vi "Power ASIC EEPROM Read.vi"(8 "error in (no error)":errorcluster) -> (0 "error out":errorcluster, 2 "results string":string, 3 "Cluster":T1)   [LabVIEW 2010]
panel:
  in  "Silicon Revision":enum16{"Rev 1-2", "Rev 3 +"}(ring)
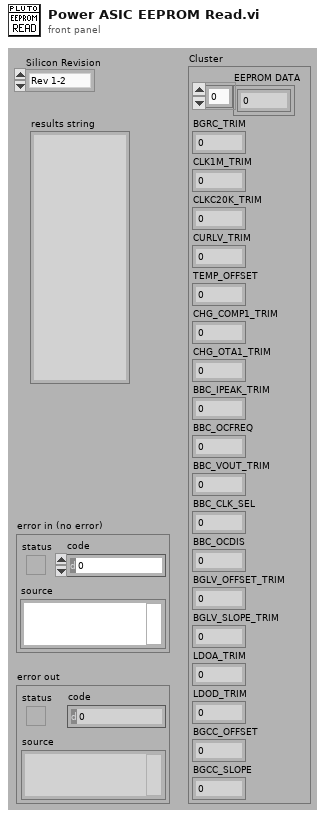
[diagram p1: front panel]
types:
  T1 = cluster{"EEPROM DATA":u32[], "BGRC_TRIM":u16, "CLK1M_TRIM":u16, "CLKC20K_TRIM":u16, "CURLV_TRIM":u16, "TEMP_OFFSET":u16, "CHG_COMP1_TRIM":u16, "CHG_OTA1_TRIM":u16, "BBC_IPEAK_TRIM":u16, "BBC_OCFREQ":u16, "BBC_VOUT_TRIM":u16, "BBC_CLK_SEL":u16, "BBC_OCDIS":u16, "BGLV_OFFSET_TRIM":u16, "BGLV_SLOPE_TRIM":u16, "LDOA_TRIM":u16, "LDOD_TRIM":u16, "BGCC_OFFSET":u16, "BGCC_SLOPE":u16}
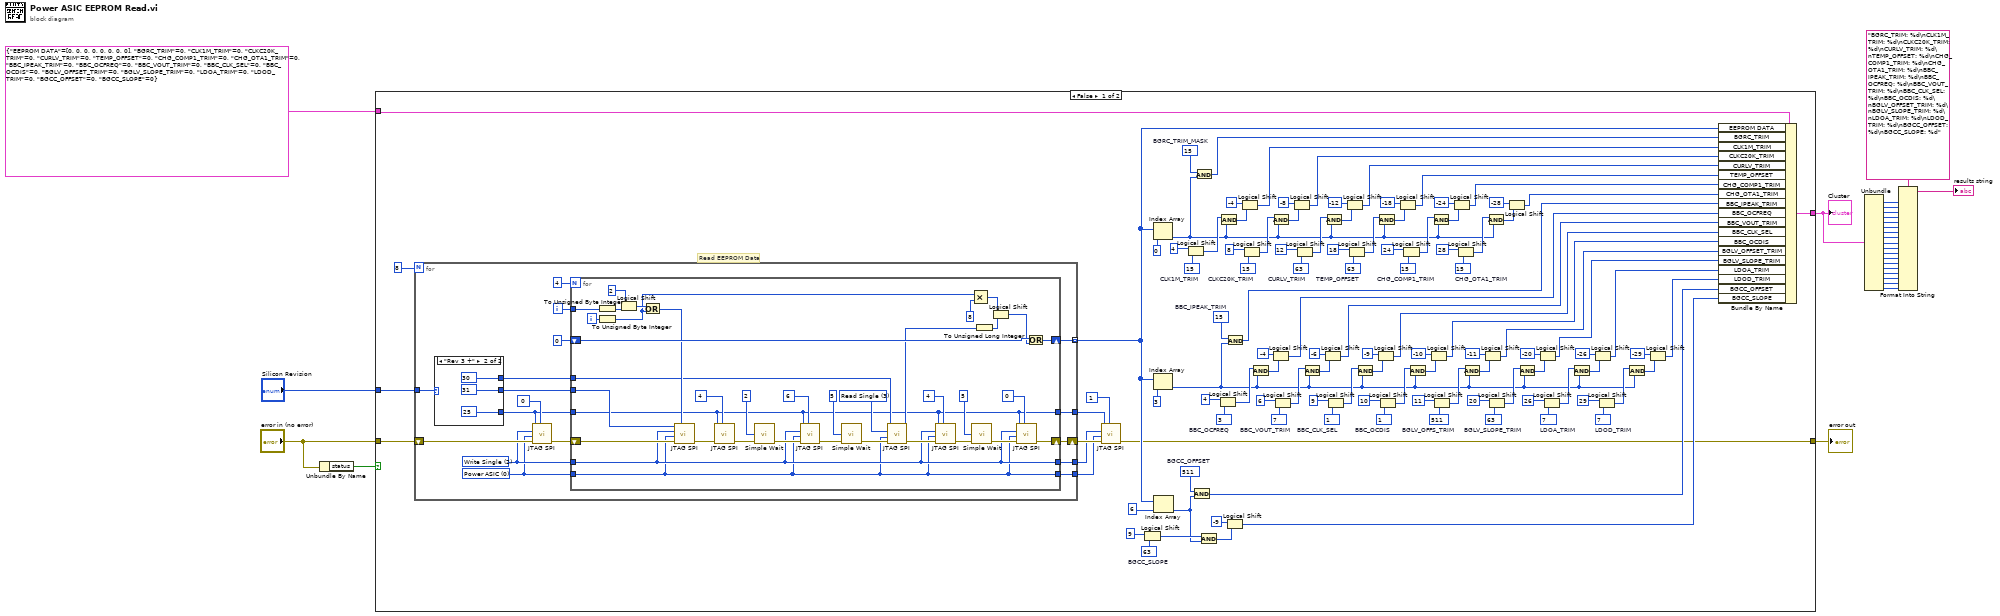
[diagram p0: block diagram]
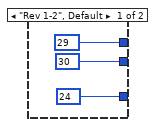
[diagram p2: hidden frame]
diagram:
  n1 = Unbundle By Name("error in (no error)") -> ("status"=w25:bool)
  n2 = case shown="False" w25 {
    tunnel: "error in (no error)" -> [w140 w201]
    tunnel: [w32 w201] -> w24
    tunnel: T1 {"EEPROM DATA"=[0, 0, 0, 0, 0, 0, 0, 0], "BGRC_TRIM"=0, "CLK1M_TRIM"=0, "CLKC20K_TRIM"=0, "CURLV_TRIM"=0, "TEMP_OFFSET"=0, "CHG_COMP1_TRIM"=0, "CHG_OTA1_TRIM"=0, "BBC_IPEAK_TRIM"=0, "BBC_OCFREQ"=0, "BBC_VOUT_TRIM"=0, "BBC_CLK_SEL"=0, "BBC_OCDIS"=0, "BGLV_OFFSET_TRIM"=0, "BGLV_SLOPE_TRIM"=0, "LDOA_TRIM"=0, "LDOD_TRIM"=0, "BGCC_OFFSET"=0, "BGCC_SLOPE"=0} -> [w135 w202]
    tunnel: [w134 w202] -> w21
    tunnel: "Silicon Revision" -> [w27 _]
    frame False {
      w36 = u32 511  # BGCC_OFFSET
      w41 = u32 63  # BGCC_SLOPE
      w60 = u32 7  # LDOD_TRIM
      w55 = u32 7  # LDOA_TRIM
      w68 = u32 63  # BGLV_SLOPE_TRIM
      w73 = u32 511  # BGLV_OFFS_TRIM
      w78 = u32 1  # BBC_OCDIS
      w83 = u32 1  # BBC_CLK_SEL
      w88 = u32 7  # BBC_VOUT_TRIM
      w93 = u32 3  # BBC_OCFREQ
      w95 = u32 15  # BBC_IPEAK_TRIM
      w104 = u32 15  # CHG_OTA1_TRIM
      w109 = u32 15  # CHG_COMP1_TRIM
      w114 = u32 63  # TEMP_OFFSET
      w119 = u32 63  # CURLV_TRIM
      w125 = u32 15  # CLKC20K_TRIM
      w132 = u32 15  # CLK1M_TRIM
      w136 = u32 15  # BGRC_TRIM_MASK
      # "Read EEPROM Data"
      n3 = for {
        N: 8 -> [_]
        shift-right: [w157] -> w33
        shift-left: w140 -> [w152]
        tunnel: [w153] -> w43 mode=indexing
        tunnel: [w144] -> w31
        tunnel: [w143] -> w29
        tunnel: [w142] -> w28
        tunnel: w27 -> [w141]
        i -> [w155]
        w148 = u16 0 items=["Power ASIC", "Stim ASIC", "MICS Radio", "FRAM"] ("Target")
        w149 = u16 2 items=["Power UP", "Power DN", "Write Single", "Read Single", "Write Block", "Read Block", "Write Masked", "Test Value"] ("Function")
        n4 = case shown="\"Rev 3 +\"" w141 {
          tunnel: [u16 30 ("SPI Address") u16 31 ("SPI Address")] -> w147
          tunnel: [u16 24 ("SPI Address") u16 25 ("SPI Address")] -> w146
          tunnel: [u16 29 ("SPI Address") u16 30 ("SPI Address")] -> w145
          frame "Rev 1-2", Default {
          }
          frame "Rev 3 +" {
          }
        }
        n5 = call "JTAG SPI.vi"("Value"=u16 0 ("SPI Address"), "error in (no error)"=w152, "Target"=w148, "Function"=w149, "Address"=w146) -> ("error out"=w151:errorcluster)  [unwired: 3 in, 3 out]
        n6 = for {
          N: 4 -> [_]
          shift-right: [w171] -> w157
          shift-left: w151 -> [w186]
          tunnel: w155 -> [w189]
          shift-right: [w197] -> w153
          shift-left: u32 0 ("EEProm Data") -> [w198]
          tunnel: w149 -> [w165]
          tunnel: w148 -> [w164]
          tunnel: w147 -> [w168]
          tunnel: w146 -> [w166]
          tunnel: w145 -> [w167]
          tunnel: [w166] -> w144
          tunnel: [w165] -> w143
          tunnel: [w164] -> w142
          i -> [w188]
          w176 = u16 3 items=["Power UP", "Power DN", "Write Single", "Read Single", "Write Block", "Read Block", "Write Masked", "Test Value"] ("Function")
          n7 = To Unsigned Byte Integer(number=w189) -> (unsigned 8bit integer=w193:u8)
          n8 = To Unsigned Byte Integer(number=w188) -> (unsigned 8bit integer=w187:u8)
          n9 = Logical Shift(y=i16 2, x=w193) -> (x << y=w199:u8)
          n10 = Or(x=w199, y=w187) -> (x .or. y?=w185:u8)
          n11 = call "JTAG SPI.vi"("Value"=w185, "error in (no error)"=w186, "Target"=w164, "Function"=w165, "Address"=w168) -> ("error out"=w182:errorcluster)  [unwired: 3 in, 3 out]
          n12 = call "JTAG SPI.vi"("Value"=u16 4 ("SPI Address"), "error in (no error)"=w182, "Address"=w166) -> ("error out"=w184:errorcluster)  [unwired: 5 in, 3 out]
          n13 = call "Simple Wait.vi"("mS"=u32 2, "error in"=w184) -> ("error out"=w180:errorcluster)  [unwired: 12 in, 1 out]
          n14 = call "JTAG SPI.vi"("Value"=u16 6 ("SPI Address"), "error in (no error)"=w180, "Target"=w164, "Function"=w165, "Address"=w166) -> ("error out"=w181:errorcluster)  [unwired: 3 in, 3 out]
          n15 = call "Simple Wait.vi"("mS"=u32 5, "error in"=w181) -> ("error out"=w178:errorcluster)  [unwired: 12 in, 1 out]
          n16 = call "JTAG SPI.vi"("error in (no error)"=w178, "Target"=w164, "Function"=w176, "Address"=w167) -> ("error out"=w174:errorcluster, "Read Value"=w177:u8)  [unwired: 4 in, 2 out]
          n17 = call "JTAG SPI.vi"("Value"=u16 4 ("SPI Address"), "error in (no error)"=w174, "Target"=w164, "Function"=w165, "Address"=w166) -> ("error out"=w175:errorcluster)  [unwired: 3 in, 3 out]
          n18 = Multiply(x=w187, y=u8 8) -> (x*y=w194:u8)
          n19 = call "Simple Wait.vi"("mS"=u32 5, "error in"=w175) -> ("error out"=w170:errorcluster)  [unwired: 12 in, 1 out]
          n20 = To Unsigned Long Integer(number=w177) -> (unsigned 32bit integer=w191:u32)
          n21 = Logical Shift(y=w194, x=w191) -> (x << y=w196:u32)
          n22 = call "JTAG SPI.vi"("Value"=u16 0 ("SPI Address"), "error in (no error)"=w170, "Target"=w164, "Function"=w165, "Address"=w166) -> ("error out"=w171:errorcluster)  [unwired: 3 in, 3 out]
          n23 = Or(x=w198, y=w196) -> (x .or. y?=w197:u32)
        }
      }
      n24 = call "JTAG SPI.vi"("Value"=u16 1 ("SPI Address"), "error in (no error)"=w33, "Target"=w28, "Function"=w29, "Address"=w31) -> ("error out"=w32:errorcluster)  [unwired: 3 in, 3 out]
      n25 = Logical Shift(y=i16 9, x=w41) -> (x << y=w40:u32)
      n26 = Index Array(array=w43, index=0) -> (element=w100:u32)
      n27 = Index Array(array=w43, index=3) -> (element=w54:u32)
      n28 = Index Array(array=w43, index=6) -> (element=w37:u32)
      n29 = Logical Shift(y=i16 4, x=w132) -> (x << y=w130:u32)
      n30 = And(x=w36, y=w37) -> (x .and. y?=w35:u32)
      n31 = And(x=w136, y=w100) -> (x .and. y?=w131:u32)
      n32 = And(x=w40, y=w37) -> (x .and. y?=w38:u32)
      n33 = Logical Shift(y=i16 4, x=w93) -> (x << y=w92:u32)
      n34 = And(x=w130, y=w100) -> (x .and. y?=w128:u32)
      n35 = Logical Shift(y=i16 -9, x=w38) -> (x << y=w34:u32)
      n36 = And(x=w95, y=w54) -> (x .and. y?=w53:u32)
      n37 = Logical Shift(y=i16 -4, x=w128) -> (x << y=w127:u32)
      n38 = Logical Shift(y=i16 8, x=w125) -> (x << y=w122:u32)
      n39 = And(x=w92, y=w54) -> (x .and. y?=w90:u32)
      n40 = Logical Shift(y=i16 -4, x=w90) -> (x << y=w52:u32)
      n41 = And(x=w122, y=w100) -> (x .and. y?=w123:u32)
      n42 = Logical Shift(y=i16 6, x=w88) -> (x << y=w85:u32)
      n43 = Logical Shift(y=i16 -8, x=w123) -> (x << y=w121:u32)
      n44 = Logical Shift(y=i16 12, x=w119) -> (x << y=w116:u32)
      n45 = And(x=w85, y=w54) -> (x .and. y?=w86:u32)
      n46 = Logical Shift(y=i16 -6, x=w86) -> (x << y=w51:u32)
      n47 = And(x=w116, y=w100) -> (x .and. y?=w117:u32)
      n48 = Logical Shift(y=i16 9, x=w83) -> (x << y=w80:u32)
      n49 = Logical Shift(y=i16 -12, x=w117) -> (x << y=w99:u32)
      n50 = Logical Shift(y=i16 18, x=w114) -> (x << y=w111:u32)
      n51 = And(x=w80, y=w54) -> (x .and. y?=w81:u32)
      n52 = Logical Shift(y=i16 -9, x=w81) -> (x << y=w50:u32)
      n53 = And(x=w111, y=w100) -> (x .and. y?=w112:u32)
      n54 = Logical Shift(y=i16 10, x=w78) -> (x << y=w75:u32)
      n55 = Logical Shift(y=i16 -18, x=w112) -> (x << y=w98:u32)
      n56 = Logical Shift(y=i16 24, x=w109) -> (x << y=w106:u32)
      n57 = And(x=w75, y=w54) -> (x .and. y?=w76:u32)
      n58 = Logical Shift(y=i16 -10, x=w76) -> (x << y=w49:u32)
      n59 = And(x=w106, y=w100) -> (x .and. y?=w107:u32)
      n60 = Logical Shift(y=i16 11, x=w73) -> (x << y=w70:u32)
      n61 = Logical Shift(y=i16 -24, x=w107) -> (x << y=w97:u32)
      n62 = Logical Shift(y=i16 28, x=w104) -> (x << y=w101:u32)
      n63 = And(x=w70, y=w54) -> (x .and. y?=w71:u32)
      n64 = Logical Shift(y=i16 -11, x=w71) -> (x << y=w48:u32)
      n65 = And(x=w101, y=w100) -> (x .and. y?=w102:u32)
      n66 = Logical Shift(y=i16 20, x=w68) -> (x << y=w65:u32)
      n67 = Logical Shift(y=i16 -28, x=w102) -> (x << y=w96:u32)
      n68 = And(x=w65, y=w54) -> (x .and. y?=w66:u32)
      n69 = Logical Shift(y=i16 -20, x=w66) -> (x << y=w47:u32)
      n70 = Logical Shift(y=i16 26, x=w55) -> (x << y=w62:u32)
      n71 = And(x=w62, y=w54) -> (x .and. y?=w63:u32)
      n72 = Logical Shift(y=i16 -26, x=w63) -> (x << y=w46:u32)
      n73 = Logical Shift(y=i16 29, x=w60) -> (x << y=w57:u32)
      n74 = And(x=w57, y=w54) -> (x .and. y?=w58:u32)
      n75 = Logical Shift(y=i16 -29, x=w58) -> (x << y=w45:u32)
      n76 = Bundle By Name(cluster=w135, "EEPROM DATA"=w43, "BGRC_TRIM"=w131, "CLK1M_TRIM"=w127, "CLKC20K_TRIM"=w121, "CURLV_TRIM"=w99, "TEMP_OFFSET"=w98, "CHG_COMP1_TRIM"=w97, "CHG_OTA1_TRIM"=w96, "BBC_IPEAK_TRIM"=w53, "BBC_OCFREQ"=w52, "BBC_VOUT_TRIM"=w51, "BBC_CLK_SEL"=w50, "BBC_OCDIS"=w49, "BGLV_OFFSET_TRIM"=w48, "BGLV_SLOPE_TRIM"=w47, "LDOA_TRIM"=w46, "LDOD_TRIM"=w45, "BGCC_OFFSET"=w35, "BGCC_SLOPE"=w34) -> (w134:T1)
    }
    frame True {
    }
  }
  "error out" <- w24
  "Cluster" <- w21
  n77 = Unbundle(w21) -> ("BGRC_TRIM"=w20:u16, "CLK1M_TRIM"=w18:u16, "CLKC20K_TRIM"=w17:u16, "CURLV_TRIM"=w16:u16, "TEMP_OFFSET"=w15:u16, "CHG_COMP1_TRIM"=w14:u16, "CHG_OTA1_TRIM"=w13:u16, "BBC_IPEAK_TRIM"=w12:u16, "BBC_OCFREQ"=w11:u16, "BBC_VOUT_TRIM"=w10:u16, "BBC_CLK_SEL"=w9:u16, "BBC_OCDIS"=w8:u16, "BGLV_OFFSET_TRIM"=w7:u16, "BGLV_SLOPE_TRIM"=w6:u16, "LDOA_TRIM"=w5:u16, "LDOD_TRIM"=w4:u16, "BGCC_OFFSET"=w3:u16, "BGCC_SLOPE"=w2:u16)  [unwired: 1 out]
  n78 = Format Into String(format string="BGRC_TRIM: %d\nCLK1M_TRIM: %d\nCLKC20K_TRIM: %d\nCURLV_TRIM: %d\nTEMP_OFFSET: %d\nCHG_COMP1_TRIM: %d\nCHG_OTA1_TRIM: %d\nBBC_IPEAK_TRIM: %d\nBBC_OCFREQ: %d\nBBC_VOUT_TRIM: %d\nBBC_CLK_SEL: %d\nBBC_OCDIS: %d\nBGLV_OFFSET_TRIM: %d\nBGLV_SLOPE_TRIM: %d\nLDOA_TRIM: %d\nLDOD_TRIM: %d\nBGCC_OFFSET: %d\nBGCC_SLOPE: %d", w20, w18, w17, w16, w15, w14, w13, w12, w11, w10, w9, w8, w7, w6, w5, w4, w3, w2) -> (resulting string=→"results string":string)  [unwired: 2 in, 1 out]
